vi "FdxExitCvi.vi"(8 "error in":errorcluster) -> (0 "error out":errorcluster)   [LabVIEW 2020, in "AIM664LV.lvlib"]
uses:
  AIM664LV.lvlib
  FdxGlobalDllPath.vi
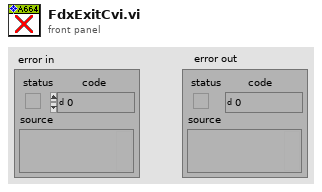
[diagram p1: front panel]
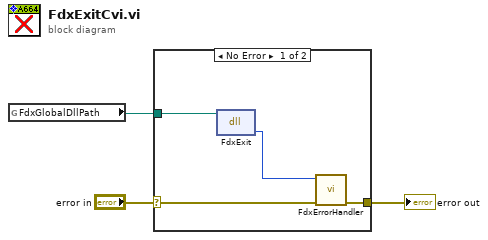
[diagram p0: block diagram]
diagram:
  n1 = global read "FdxGlobalDllPath.vi" "FdxGlobalDllPath"() -> (w1:path)
  n2 = case shown="No Error" "error in" {
    selector: "error in" -> [w6 w8]
    tunnel: [w7 w8] -> w3
    tunnel: w1 -> [w4 _]
    frame No Error {
      n3 = dll-call lib="aim_fdx.19.dll" fn="FdxExit"(path in=w4) -> ("status"=w5:i32)  [unwired: 2 in, 2 out]
      n4 = call "FdxErrorHandler.vi"("error in"=w6, "AIM Error"=w5) -> ("error out"=w7:errorcluster)  [unwired: 9 in]
    }
    frame Error {
    }
  }
  "error out" <- w3
